vi "Config.vi"(8 "error in (no error)":errorcluster, 10 "Setting":T1={"Max. Volt"=10.0, "Current Limit"=0.5, "Volt Level"=10.0}, 11 "Keysight 6700C in":refnum<class "Keysight 6700C.lvclass">) -> (0 "error out":errorcluster, 3 "Keysight 6700C out":refnum<class "Keysight 6700C.lvclass">)   [LabVIEW 2019, in "Concrete.lvlib" / "Keysight 6700C.lvclass"]
uses:
  Keysight 6700C.lvclass
  Keysight 6700C.lvclass/Keysight 6700C.ctl
  <instrlib>/Agilent N6700/Agilent N6700 Series.lvlib
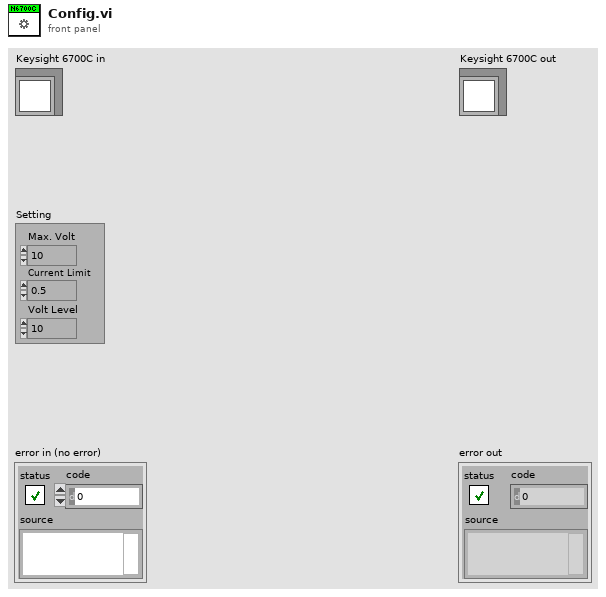
[diagram p1: front panel]
types:
  T1 = cluster{"Max. Volt":dbl, "Current Limit":dbl, "Volt Level":dbl}
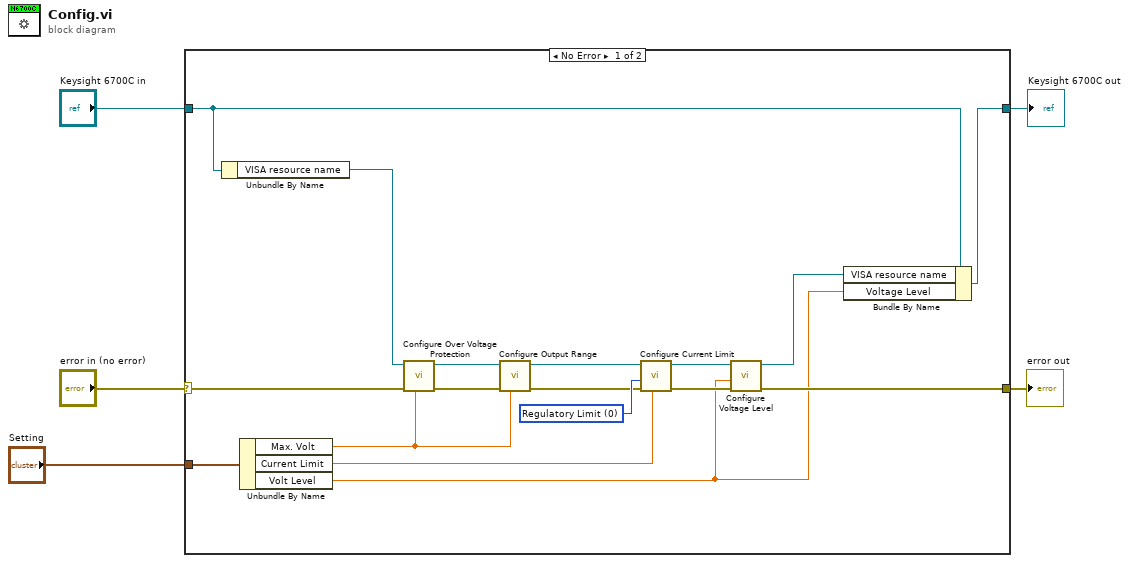
[diagram p0: block diagram]
diagram:
  n1 = case shown="No Error" "error in (no error)" {
    selector: "error in (no error)" -> [w18 w24]
    tunnel: [w8 w24] -> w4
    tunnel: [w19 w23] -> w2
    tunnel: "Keysight 6700C in" -> [w20 w23]
    tunnel: "Setting" -> [w21 _]
    frame No Error {
      w22 = 0 items=["Regulatory Limit", "Trip Limit"] ("Behavior (0: Regulatory Limit)")
      n2 = Unbundle By Name(w20) -> ("VISA resource name"=w17:refnum<visa-resource-name>)
      n3 = Unbundle By Name(w21) -> ("Max. Volt"=w14:dbl, "Current Limit"=w13:dbl, "Volt Level"=w7:dbl)
      n4 = call <instrlib>:"Configure Over Voltage Protection.vi"("Limit (0.0 volts)"=w14, "error in (no error)"=w18, "VISA resource name"=w17) -> ("error out"=w16:errorcluster, "VISA resource name out"=w15:refnum<visa-resource-name>)  [unwired: 7 in]
      n5 = call <instrlib>:"Configure Output Range.vi"("Range (0.0)"=w14, "error in (no error)"=w16, "VISA resource name"=w15) -> ("error out"=w12:errorcluster, "VISA resource name out"=w11:refnum<visa-resource-name>)  [unwired: 7 in]
      n6 = call <instrlib>:"Configure Current Limit.vi"("Limit (0.0 amps)"=w13, "error in (no error)"=w12, "Behavior (0: Regulatory Limit)"=w22, "VISA resource name"=w11) -> ("error out"=w10:errorcluster, "VISA resource name out"=w9:refnum<visa-resource-name>)  [unwired: 6 in]
      n7 = call <instrlib>:"Configure Voltage Level.vi"("error in (no error)"=w10, "Level  (0.0 volts)"=w7, "VISA resource name"=w9) -> ("error out"=w8:errorcluster, "VISA resource name out"=w6:refnum<visa-resource-name>)  [unwired: 7 in]
      n8 = Bundle By Name(cluster=w20, "VISA resource name"=w6, "Voltage Level"=w7) -> (w19:refnum<class "Keysight 6700C.lvclass">)
    }
    frame Error {
    }
  }
  "error out" <- w4
  "Keysight 6700C out" <- w2
